vi "PH_Connection.get PSDB.vi"(2 "error in (no error)":errorcluster) -> (0 "error out":errorcluster, 1 "PSDB Credentials":T1={"PW"="N/A", "ID"="N/A", "DS"="N/A"})   [LabVIEW 2014, in "PH_Common.lvlib"]
uses:
  PH_Common.lvlib
  PH_Connection.PSDB Credentials.ctl
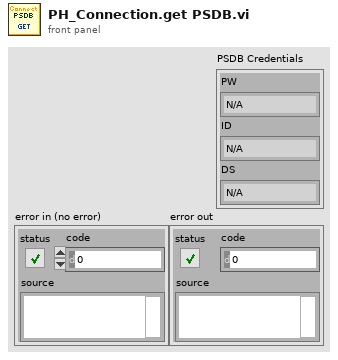
[diagram p1: front panel]
types:
  T1 = typedef "PH_Common.lvlib/PH_Connection.PSDB Credentials.ctl" = cluster{"PW":string, "ID":string, "DS":string}
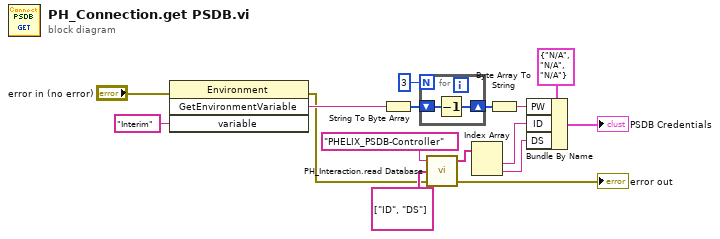
[diagram p0: block diagram]
diagram:
  n1 = invoke class="Environment" method="GetEnvironmentVariable"(error in="error in (no error)", "variable"="Interim") -> (error out=w3:errorcluster, "GetEnvironmentVariable"=w7:string)  [unwired: 2 in, 2 out]
  n2 = String To Byte Array(string=w7) -> (unsigned byte array=w15:u8[])
  n3 = for {
    N: 3 -> [_]
    shift-right: [w17] -> w14
    shift-left: w15 -> [w18]
    n4 = Decrement(x=w18) -> (x-1=w17:u8[])
  }
  n5 = call "PH_Interaction.read Database.vi"("error in (no error)"=w3, "Strings to search for"=string[] ["ID", "DS"], "DB Entry to read"="PHELIX_PSDB-Controller") -> ("error out"=→"error out":errorcluster, "Values"=w12:string[])  [unwired: 1 in]
  n6 = Index Array(array=w12) -> (element #1=w5:string, element #2=w4:string)  [unwired: 2 in]
  n7 = Byte Array To String(unsigned byte array=w14) -> (string=w6:string)
  n8 = Bundle By Name(cluster=T1 {"PW"="N/A", "ID"="N/A", "DS"="N/A"} ("PSDB Credentials"), "PW"=w6, "ID"=w5, "DS"=w4) -> (→"PSDB Credentials":T1)
